vi "Export - UDP Custom Device.vi"(8 "error in (no error)":errorcluster, 10 "Target File":path, 11 "Device Item Ref in":T1 format="%.0x") -> (0 "error out":errorcluster)   [LabVIEW 2016, in "UDP-Custom-Device System Explorer.lvlib"]
uses:
  UDP-Custom-Device System Explorer.lvlib
  <vilib>/NI Veristand/Custom Device API/Custom Device Item Ref.ctl
  <vilib>/NI VeriStand/Custom Device API/Custom Device API.lvlib
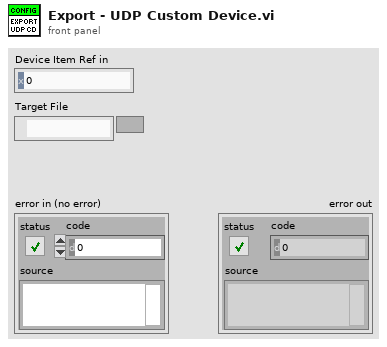
[diagram p1: front panel]
types:
  T1 = typedef "Custom Device API.lvlib/Custom Device Item Ref.ctl" = u64
  T2 = typedef "UDP-Custom-Device System Explorer.lvlib/ImpExp - Data.ctl" = cluster{"Import/Export Data - Main":T3, "Rx Packets":T5, "Tx Packets":T8}
  T3 = typedef "UDP-Custom-Device System Explorer.lvlib/ImpExp - Main Data.ctl" = cluster{"Common":T4, "Export File Location":path, "Export to File Status":bool, "Timestamp Path":string, "Description":string}
  T4 = typedef "Custom Device API.lvlib/Custom Device Item Info.ctl" = cluster{"Name":string, "Is Channel":bool, "GUID":string, "Is Waveform":bool}
  T5 = typedef "UDP-Custom-Device System Explorer.lvlib/ImpExp - Rx Packets Data.ctl" = cluster{"Common":T4, "Packet Names":string[], "Packet IDs":i32[], "Packet Paths":string[], "Rx Packet Data":T6[]}
  T6 = typedef "UDP-Custom-Device System Explorer.lvlib/ImpExp - Rx Packet Data.ctl" = cluster{"Common":T4, "Packet ID":i32, "Header Info":u32, "Auto-Assign NIC":bool, "IP Address of Local NIC":string, "Port":u16, "Read Timeout":i32, "Endianness":u16, "Channel Names":string[], "Data Types":T7[], "Description":string}
  T7 = typedef "UDP-Custom-Device Shared.lvlib/Shared - Channel Data Type.ctl" = enum16{"Boolean", "Single", "Double", "I8", "I16", "I32", "I64", "U8", "U16", "U32", "U64"}
  T8 = typedef "UDP-Custom-Device System Explorer.lvlib/ImpExp - Tx Packets Data.ctl" = cluster{"Common":T4, "Packet IDs":i32[], "Packet Names":string[], "Packet Paths":string[], "Tx Packet Data":T9[]}
  T9 = typedef "UDP-Custom-Device System Explorer.lvlib/ImpExp - Tx Packet Data.ctl" = cluster{"Common":T4, "Packet ID":i32, "Header Info":u32, "Auto-Assign NIC":bool, "IP Address of Local NIC":string, "Port":u16, "Destination IP":string, "Destination Port":u16, "Endianness":u16, "Decimation":u16, "Channel Names":string[], "Channel Paths":string[], "Data types":T7[], "Timestamp Path":string, "Description":string}
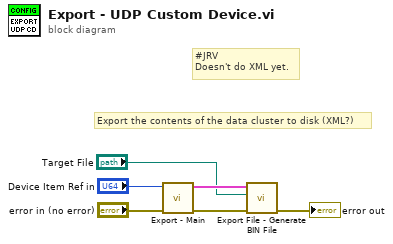
[diagram p0: block diagram]
diagram:
  # "#JRV\nDoesn't do XML yet."
  # "Export the contents of the data cluster to disk (XML?)"
  n1 = call "Export - Main.vi"("error in (no error)"="error in (no error)", "Device Item Ref in"="Device Item Ref in") -> ("error out"=w2:errorcluster, "Import/Export Data"=w4:T2)  [unwired: 8 in]
  n2 = call "Export File - Generate BIN File.vi"("error in (no error)"=w2, "Target File"="Target File", "Import/Export Data"=w4) -> ("error out"=→"error out":errorcluster)  [unwired: 8 in]
